vi "main.vi"() -> ()   [LabVIEW 2017]
uses:
  <vilib>/Utility/miscctls.llb/LVRectTypeDef.ctl
  Str_Lam&Sil.ctl
panel:
  out "Wjazd z obu stron":bool
  out "Ilość samochodów na parkingu":dbl
  out "Aktualny stan":T1(ring)
  out "Która brama pierwsza":enum16{"Nikt", "Brama 1", "Brama 2"}(ring)
  in  "output cluster":T2
  out "Brama 2 - kto pierwszy":T3(ring)
  out "Brama 1 - kto pierwszy":T3(ring)
  in  "Ilość miejsc na parkingu":dbl=4.0
  in  "stop":bool
  in  "Dane in":T4
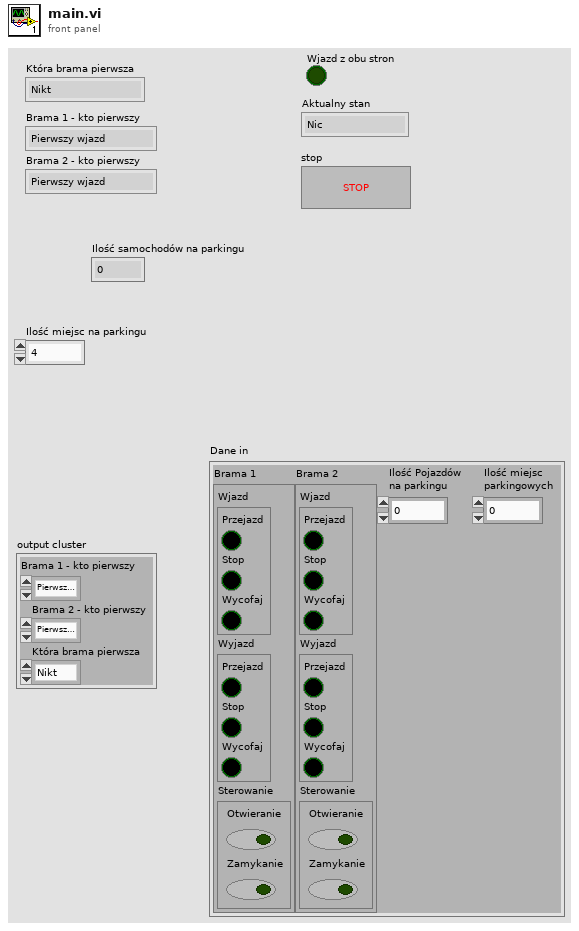
[diagram p1: front panel]
types:
  T1 = enum16{"Nic", "Otwieranie", "Otwarte", "Wjazd", "Wyjazd", "Zamykanie", "Wycofaj", "Blad"}
  T2 = cluster{"Brama 1 - kto pierwszy":enum16{"Pierwszy wjazd", "Nikt", "Pierwszy wyjazd"}, "Brama 2 - kto pierwszy":enum16{"Pierwszy wjazd", "Nikt", "Pierwszy wyjazd"}, "Która brama pierwsza":enum16{"Nikt", "Brama 1", "Brama 2"}}
  T3 = enum16{"Pierwszy wjazd", "Nikt", "Pierwszy wyjazd"}
  T4 = cluster{"Brama 1":cluster{"Wjazd":cluster{"Wjazd Przejazd":bool, "Wjazd Stop":bool, "Wjazd Wycofaj":bool}, "Wyjazd":cluster{"Wjazd Przejazd":bool, "Wjazd Stop":bool, "Wjazd Wycofaj":bool}, "Sterowanie":cluster{"Otwieranie":bool, "Zamykanie":bool}}, "Brama 2":cluster{"Wjazd":cluster{"Wjazd Przejazd":bool, "Wjazd Stop":bool, "Wjazd Wycofaj":bool}, "Wyjazd":cluster{"Wjazd Przejazd":bool, "Wjazd Stop":bool, "Wjazd Wycofaj":bool}, "Sterowanie":cluster{"Otwieranie":bool, "Zamykanie":bool}}, "Ilość Pojazdów \nna parkingu":dbl, "Ilość miejsc \nparkingowych":dbl}
  T5 = typedef "LVRectTypeDef.ctl" = cluster{"Left":i16, "Top":i16, "Right":i16, "Bottom":i16}
  T6 = typedef "Str_Lam&Sil.ctl" = bool
  T7 = cluster{"Wjazd":cluster{"Wjazd Przejazd":T6, "Wjazd Stop":bool, "Wjazd Wycofaj":bool}, "Wyjazd":cluster{"Wjazd Przejazd":bool, "Wjazd Stop":bool, "Wjazd Wycofaj":bool}, "Sterowanie":cluster{"Otwieranie":bool, "Zamykanie":bool}}
  T8 = cluster{"czujnik laserowy \nwjazd":bool, "czujnik laserowy wyjazd":bool, "czujnik laserowy \nbrama zamknięta":bool, "czujnik laserowy \nbrama otwarta":bool}
  T9 = cluster{"Brama 1":cluster{"czujnik laserowy \nwjazd":bool, "czujnik laserowy wyjazd":bool, "czujnik laserowy \nbrama zamknięta":bool, "czujnik laserowy \nbrama otwarta":bool}, "Brama 2":cluster{"czujnik laserowy \nwjazd":bool, "czujnik laserowy wyjazd":bool, "czujnik laserowy \nbrama zamknięta":bool, "czujnik laserowy \nbrama otwarta":bool}}
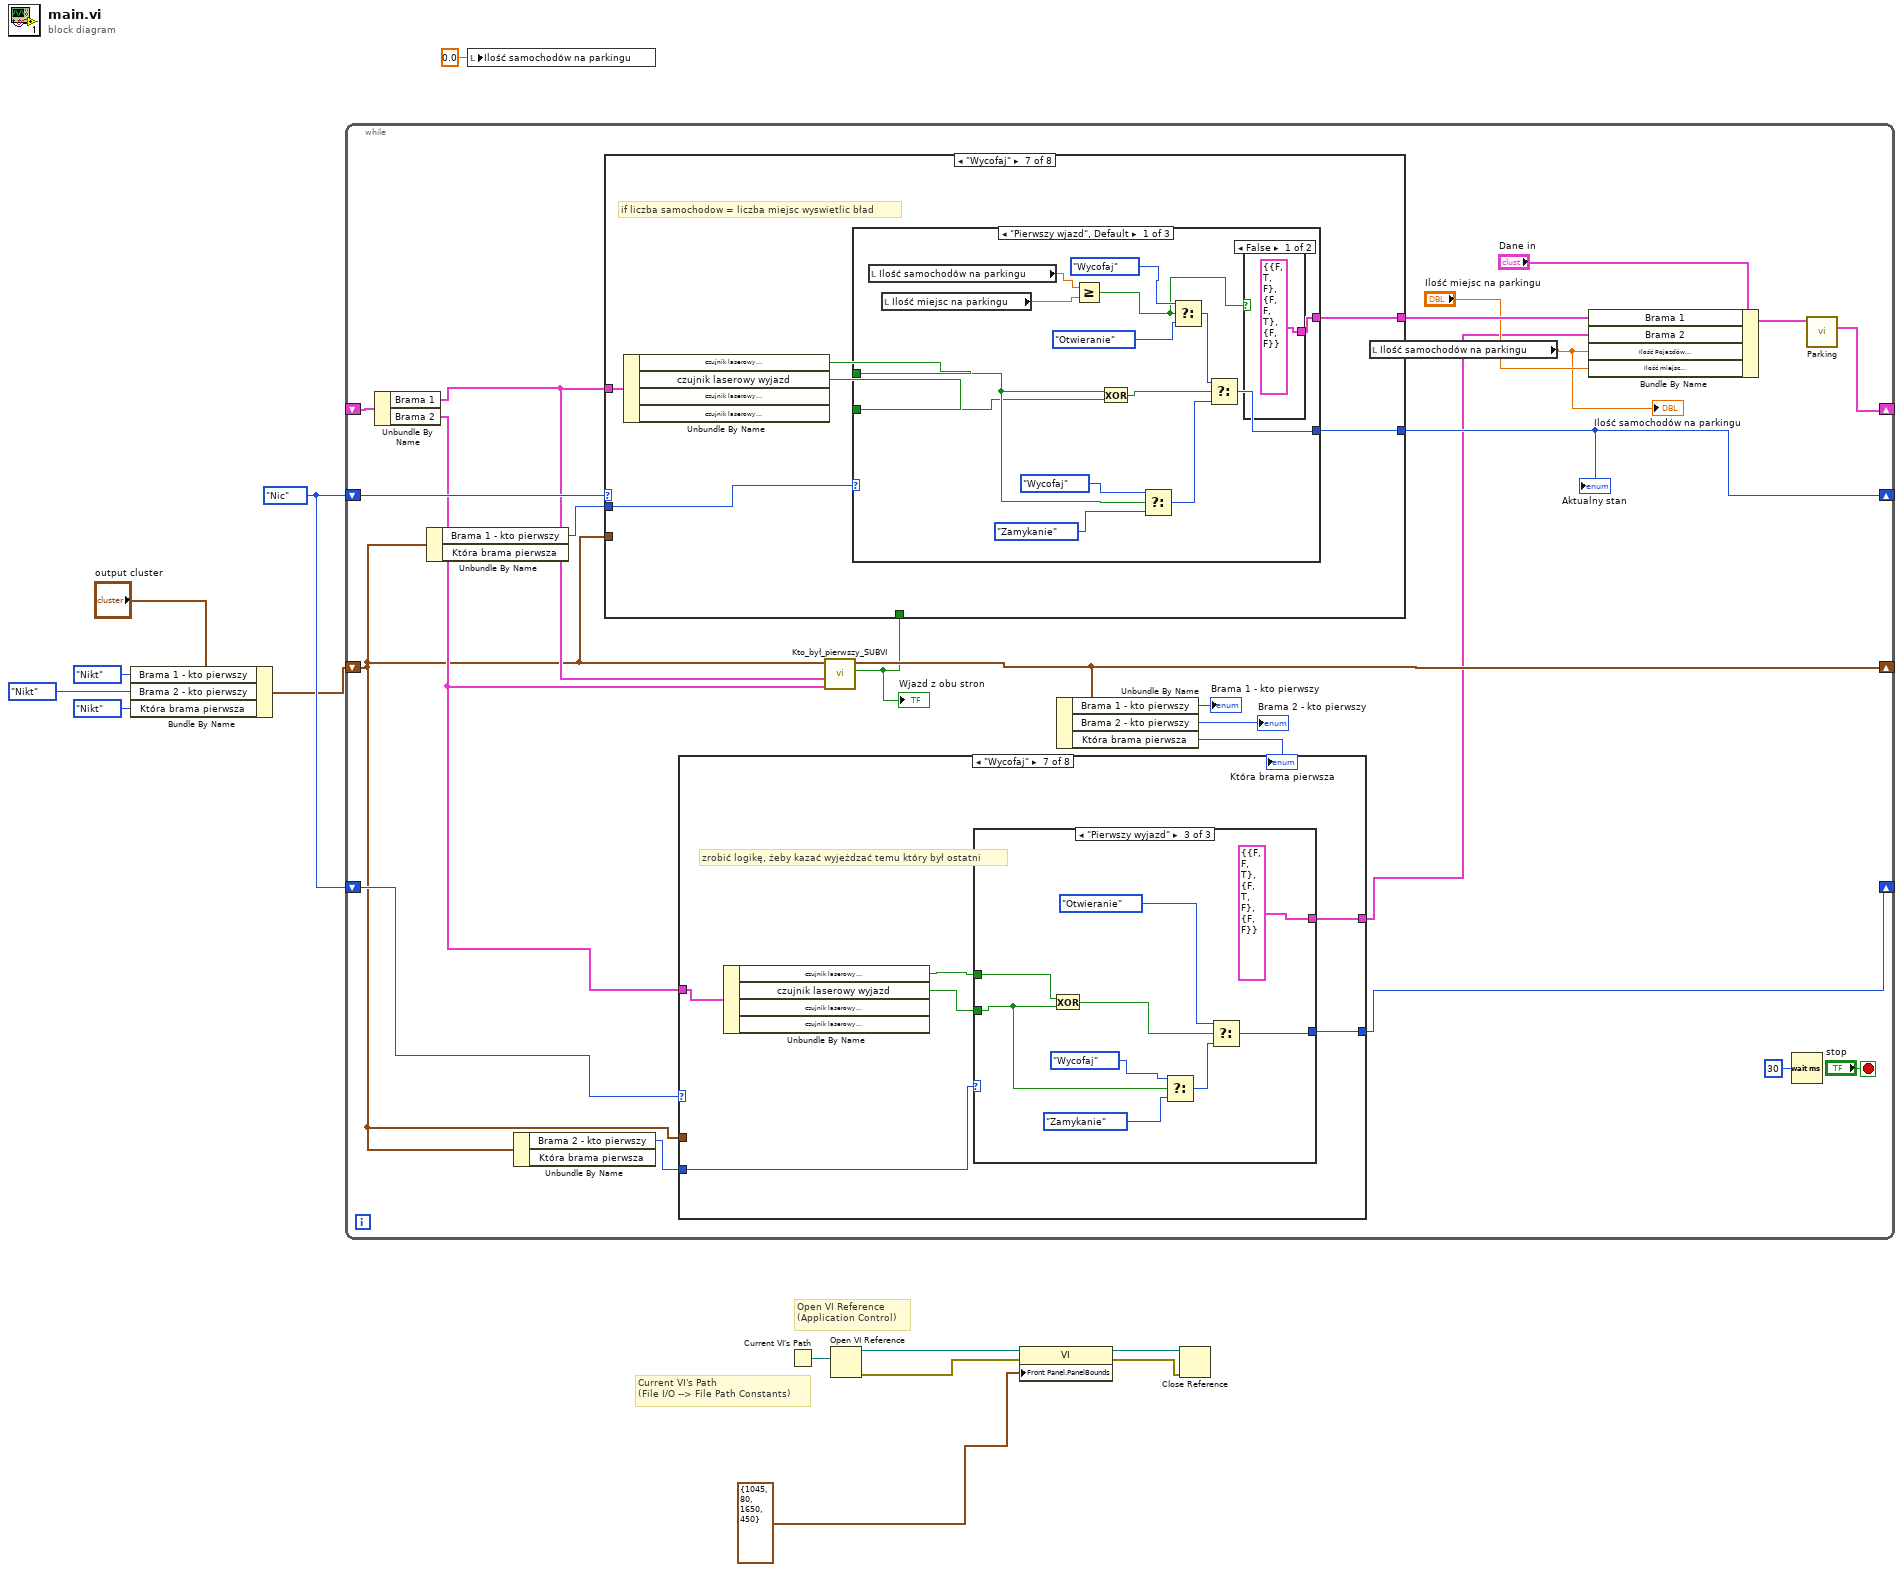
[diagram p0: block diagram]
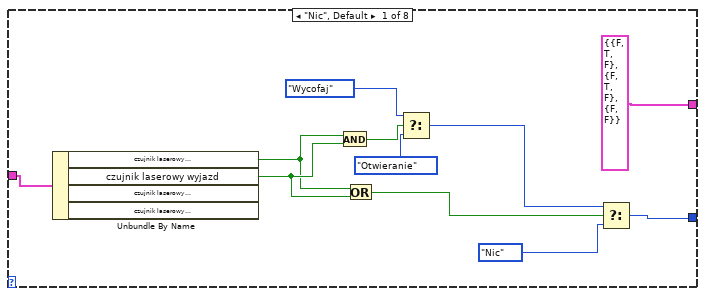
[diagram p2: hidden frame]
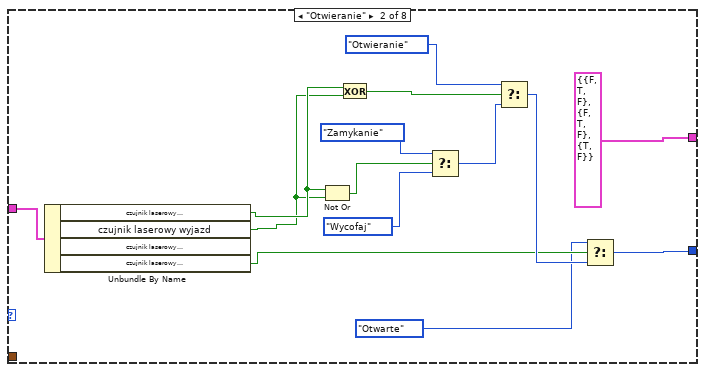
[diagram p3: hidden frame]
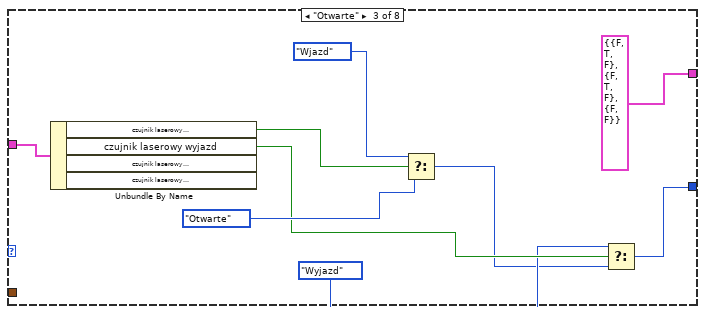
[diagram p4: hidden frame]
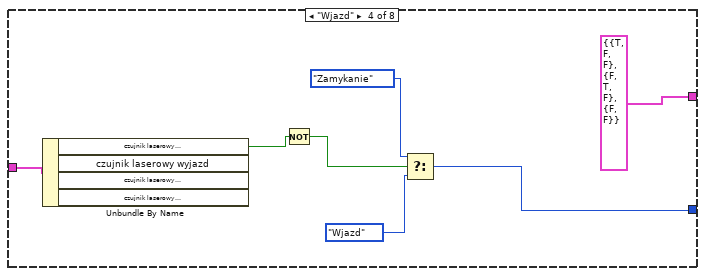
[diagram p5: hidden frame]
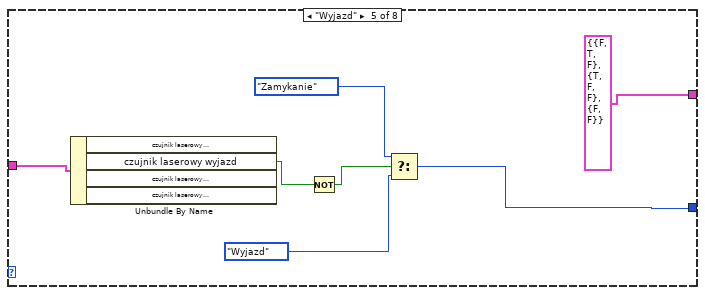
[diagram p6: hidden frame]
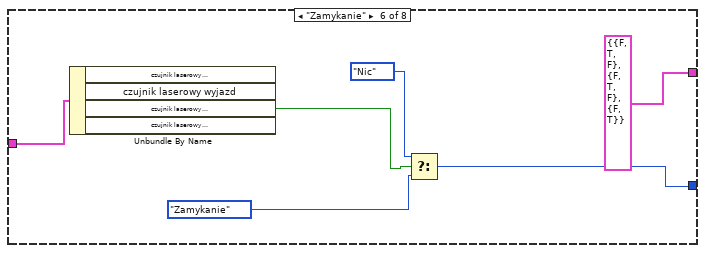
[diagram p7: hidden frame]
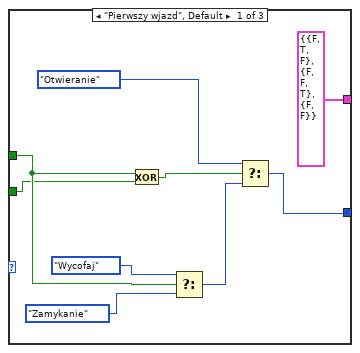
[diagram p8: hidden frame]
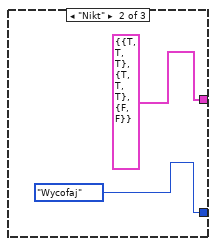
[diagram p9: hidden frame]
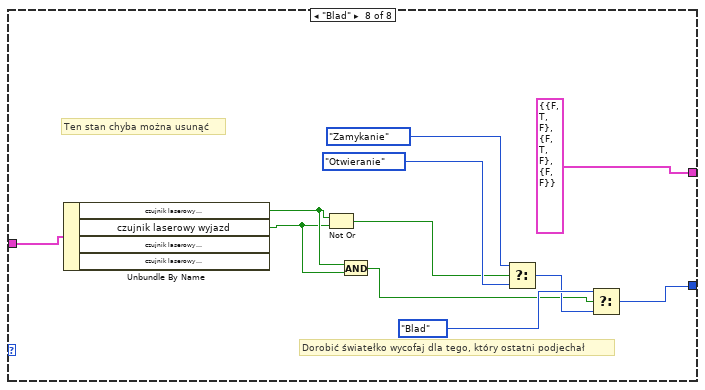
[diagram p10: hidden frame]
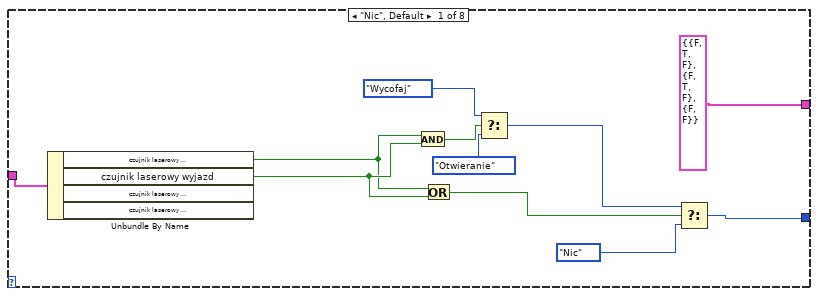
[diagram p11: hidden frame]
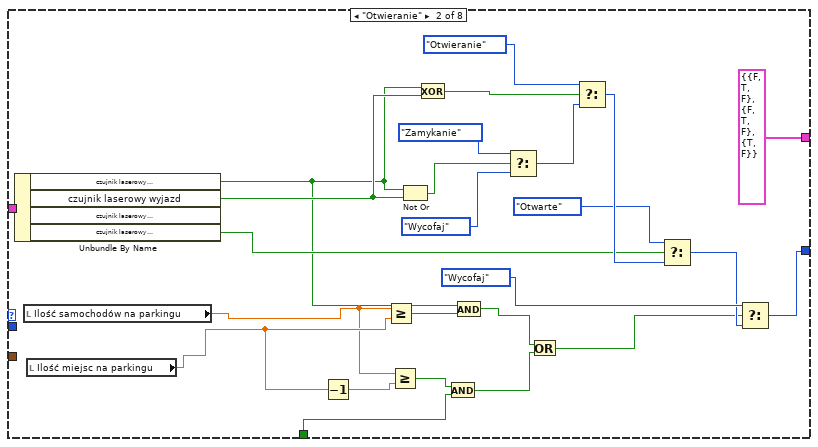
[diagram p12: hidden frame]
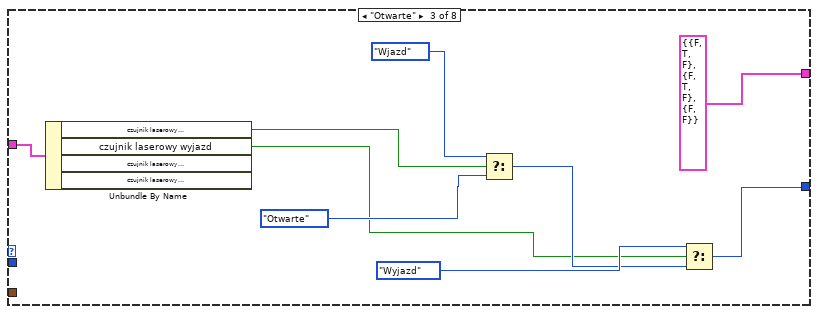
[diagram p13: hidden frame]
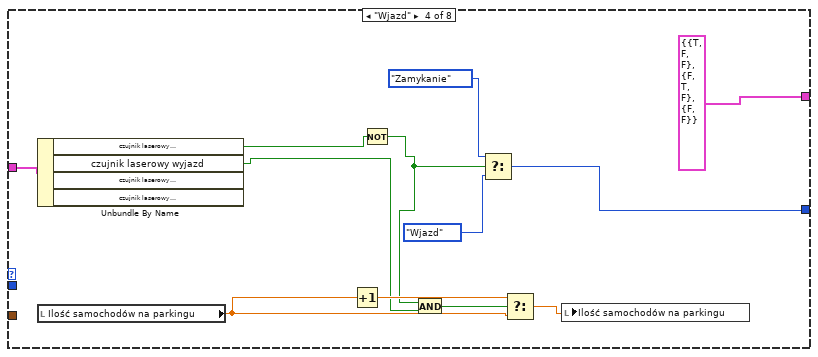
[diagram p14: hidden frame]
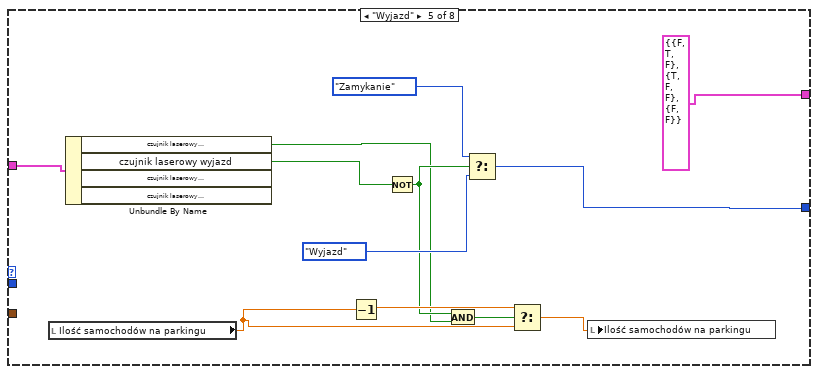
[diagram p15: hidden frame]
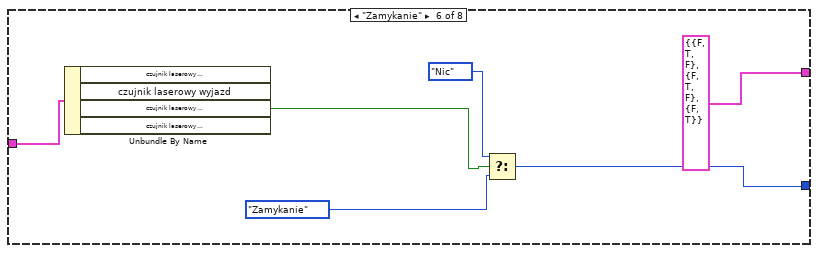
[diagram p16: hidden frame]
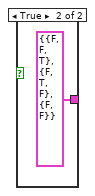
[diagram p17: hidden frame]
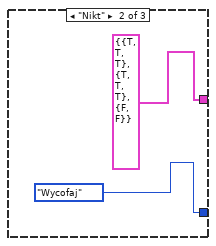
[diagram p18: hidden frame]
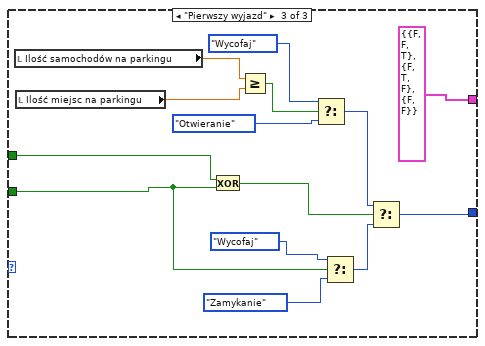
[diagram p19: hidden frame]
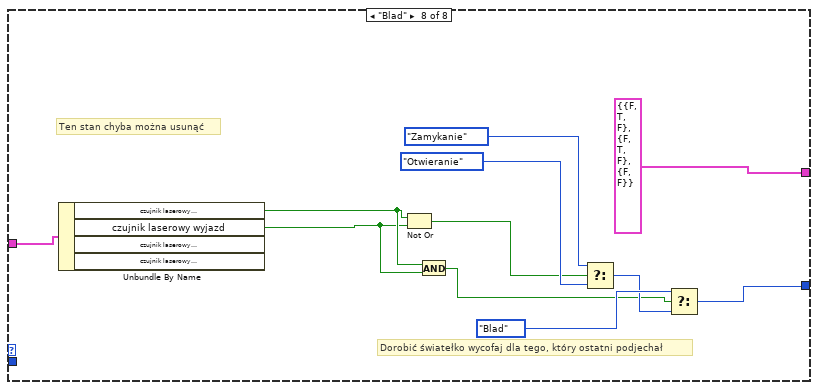
[diagram p20: hidden frame]
diagram:
  w13 = T1."Nic"
  # "Open VI Reference\n(Application Control)"
  # "Current VI's Path\n(File I/O --> File Path Constants)"
  n1 = Bundle By Name(cluster="output cluster", "Brama 1 - kto pierwszy"=T3."Nikt", "Brama 2 - kto pierwszy"=T3."Nikt", "Która brama pierwsza"=enum16{"Nikt", "Brama 1", "Brama 2"}."Nikt") -> (w11:T2)
  n2 = while {
    shift-right: [w34] -> _
    shift-left: _ -> [w35]
    shift-right: [w31] -> _
    shift-left: w13 -> [w29]
    shift-right: [w21] -> _
    shift-left: w13 -> [w20]
    shift-right: [w26] -> _
    shift-left: w11 -> [w18]
    stop <- "stop" stop-if-true
    n3 = Unbundle By Name(w35) -> ("Brama 1"=w27:T8, "Brama 2"=w19:T8)
    n4 = Unbundle By Name(w18) -> ("Brama 1 - kto pierwszy"=w16:T3)  [unwired: 1 out]
    n5 = Unbundle By Name(w18) -> ("Brama 2 - kto pierwszy"=w15:T3)  [unwired: 1 out]
    n6 = case shown="\"Wycofaj\"" w20 {
      tunnel: w19 -> [w40 w62 w63 w76 w81 w88 w97 w127]
      tunnel: [w41 w61 w65 w75 w83 w86 w93 w124] -> w21
      tunnel: [T7 {"Wjazd"={"Wjazd Przejazd"=FALSE, "Wjazd Stop"=TRUE, "Wjazd Wycofaj"=FALSE}, "Wyjazd"={"Wjazd Przejazd"=FALSE, "Wjazd Stop"=TRUE, "Wjazd Wycofaj"=FALSE}, "Sterowanie"={"Otwieranie"=FALSE, "Zamykanie"=FALSE}} ("Brama 1") T7 {"Wjazd"={"Wjazd Przejazd"=FALSE, "Wjazd Stop"=TRUE, "Wjazd Wycofaj"=FALSE}, "Wyjazd"={"Wjazd Przejazd"=FALSE, "Wjazd Stop"=TRUE, "Wjazd Wycofaj"=FALSE}, "Sterowanie"={"Otwieranie"=TRUE, "Zamykanie"=FALSE}} ("Brama 1") T7 {"Wjazd"={"Wjazd Przejazd"=FALSE, "Wjazd Stop"=TRUE, "Wjazd Wycofaj"=FALSE}, "Wyjazd"={"Wjazd Przejazd"=FALSE, "Wjazd Stop"=TRUE, "Wjazd Wycofaj"=FALSE}, "Sterowanie"={"Otwieranie"=FALSE, "Zamykanie"=FALSE}} ("Brama 1") T7 {"Wjazd"={"Wjazd Przejazd"=TRUE, "Wjazd Stop"=FALSE, "Wjazd Wycofaj"=FALSE}, "Wyjazd"={"Wjazd Przejazd"=FALSE, "Wjazd Stop"=TRUE, "Wjazd Wycofaj"=FALSE}, "Sterowanie"={"Otwieranie"=FALSE, "Zamykanie"=FALSE}} ("Brama 1") T7 {"Wjazd"={"Wjazd Przejazd"=FALSE, "Wjazd Stop"=TRUE, "Wjazd Wycofaj"=FALSE}, "Wyjazd"={"Wjazd Przejazd"=TRUE, "Wjazd Stop"=FALSE, "Wjazd Wycofaj"=FALSE}, "Sterowanie"={"Otwieranie"=FALSE, "Zamykanie"=FALSE}} ("Brama 1") T7 {"Wjazd"={"Wjazd Przejazd"=FALSE, "Wjazd Stop"=TRUE, "Wjazd Wycofaj"=FALSE}, "Wyjazd"={"Wjazd Przejazd"=FALSE, "Wjazd Stop"=TRUE, "Wjazd Wycofaj"=FALSE}, "Sterowanie"={"Otwieranie"=FALSE, "Zamykanie"=TRUE}} ("Brama 1") w94 T7 {"Wjazd"={"Wjazd Przejazd"=FALSE, "Wjazd Stop"=TRUE, "Wjazd Wycofaj"=FALSE}, "Wyjazd"={"Wjazd Przejazd"=FALSE, "Wjazd Stop"=TRUE, "Wjazd Wycofaj"=FALSE}, "Sterowanie"={"Otwieranie"=FALSE, "Zamykanie"=FALSE}} ("Brama 1")] -> w22
      tunnel: w18 -> [_ _ _ _ _ _ _ _]
      tunnel: w15 -> [_ _ _ _ _ _ w92 _]
      frame "Nic", Default {
        n7 = Unbundle By Name(w40) -> ("czujnik laserowy \nwjazd"=w38:bool, "czujnik laserowy wyjazd"=w46:bool)  [unwired: 2 out]
        n8 = And(x=w38, y=w46) -> (x .and. y?=w48:bool)
        n9 = Or(x=w38, y=w46) -> (x .or. y?=w45:bool)
        n10 = Select(t=T1."Wycofaj", s=w48, f=T1."Otwieranie") -> (s? t:f=w44:T1)
        n11 = Select(t=w44, s=w45, f=T1."Nic") -> (s? t:f=w41:T1)
      }
      frame "Otwieranie" {
        n12 = Unbundle By Name(w62) -> ("czujnik laserowy \nwjazd"=w52:bool, "czujnik laserowy wyjazd"=w51:bool, "czujnik laserowy \nbrama otwarta"=w58:bool)  [unwired: 1 out]
        n13 = Not Or(1:w51, 2:w52) -> (0:w56:bool)
        n14 = Exclusive Or(1:w51, 2:w52) -> (0:w53:bool)
        n15 = Select(t=T1."Zamykanie", s=w56, f=T1."Wycofaj") -> (s? t:f=w49:T1)
        n16 = Select(t=T1."Otwieranie", s=w53, f=w49) -> (s? t:f=w59:T1)
        n17 = Select(t=T1."Otwarte", s=w58, f=w59) -> (s? t:f=w61:T1)
      }
      frame "Otwarte" {
        n18 = Unbundle By Name(w63) -> ("czujnik laserowy \nwjazd"=w69:bool, "czujnik laserowy wyjazd"=w68:bool)  [unwired: 2 out]
        n19 = Select(t=T1."Wjazd", s=w69, f=T1."Otwarte") -> (s? t:f=w66:T1)
        n20 = Select(t=T1."Wyjazd", s=w68, f=w66) -> (s? t:f=w65:T1)
      }
      frame "Wjazd" {
        n21 = Unbundle By Name(w76) -> ("czujnik laserowy \nwjazd"=w73:bool)  [unwired: 3 out]
        n22 = Not(x=w73) -> (.not. x?=w72:bool)
        n23 = Select(t=T1."Zamykanie", s=w72, f=T1."Wjazd") -> (s? t:f=w75:T1)
      }
      frame "Wyjazd" {
        n24 = Unbundle By Name(w81) -> ("czujnik laserowy wyjazd"=w80:bool)  [unwired: 3 out]
        n25 = Not(x=w80) -> (.not. x?=w79:bool)
        n26 = Select(t=T1."Zamykanie", s=w79, f=T1."Wyjazd") -> (s? t:f=w83:T1)
      }
      frame "Zamykanie" {
        n27 = Unbundle By Name(w88) -> ("czujnik laserowy \nbrama zamknięta"=w87:bool)  [unwired: 3 out]
        n28 = Select(t=T1."Nic", s=w87, f=T1."Zamykanie") -> (s? t:f=w86:T1)
      }
      frame "Wycofaj" {
        # "zrobić logikę, żeby kazać wyjeżdzać temu który był ostatni"
        n29 = Unbundle By Name(w97) -> ("czujnik laserowy \nwjazd"=w95:bool, "czujnik laserowy wyjazd"=w96:bool)  [unwired: 2 out]
        n30 = case shown="\"Pierwszy wyjazd\"" w92 {
          tunnel: w96 -> [w98 _ w109]
          tunnel: w95 -> [w99 _ w115]
          tunnel: [T7 {"Wjazd"={"Wjazd Przejazd"=FALSE, "Wjazd Stop"=TRUE, "Wjazd Wycofaj"=FALSE}, "Wyjazd"={"Wjazd Przejazd"=FALSE, "Wjazd Stop"=FALSE, "Wjazd Wycofaj"=TRUE}, "Sterowanie"={"Otwieranie"=FALSE, "Zamykanie"=FALSE}} ("Brama 1") T7 {"Wjazd"={"Wjazd Przejazd"=TRUE, "Wjazd Stop"=TRUE, "Wjazd Wycofaj"=TRUE}, "Wyjazd"={"Wjazd Przejazd"=TRUE, "Wjazd Stop"=TRUE, "Wjazd Wycofaj"=TRUE}, "Sterowanie"={"Otwieranie"=FALSE, "Zamykanie"=FALSE}} ("Brama 1") T7 {"Wjazd"={"Wjazd Przejazd"=FALSE, "Wjazd Stop"=FALSE, "Wjazd Wycofaj"=TRUE}, "Wyjazd"={"Wjazd Przejazd"=FALSE, "Wjazd Stop"=TRUE, "Wjazd Wycofaj"=FALSE}, "Sterowanie"={"Otwieranie"=FALSE, "Zamykanie"=FALSE}} ("Brama 1")] -> w94
          tunnel: [w104 T1."Wycofaj" w116] -> w93
          frame "Pierwszy wjazd", Default {
            n31 = Exclusive Or(1:w98, 2:w99) -> (0:w100:bool)
            n32 = Select(t=T1."Wycofaj", s=w99, f=T1."Zamykanie") -> (s? t:f=w101:T1)
            n33 = Select(t=T1."Otwieranie", s=w100, f=w101) -> (s? t:f=w104:T1)
          }
          frame "Nikt" {
          }
          frame "Pierwszy wyjazd" {
            n34 = Exclusive Or(1:w109, 2:w115) -> (0:w114:bool)
            n35 = Select(t=T1."Wycofaj", s=w109, f=T1."Zamykanie") -> (s? t:f=w110:T1)
            n36 = Select(t=T1."Otwieranie", s=w114, f=w110) -> (s? t:f=w116:T1)
          }
        }
      }
      frame "Blad" {
        # "Ten stan chyba można usunąć"
        # "Dorobić światełko wycofaj dla tego, który ostatni podjechał"
        n37 = Unbundle By Name(w127) -> ("czujnik laserowy \nwjazd"=w120:bool, "czujnik laserowy wyjazd"=w119:bool)  [unwired: 2 out]
        n38 = Not Or(1:w119, 2:w120) -> (0:w121:bool)
        n39 = And(x=w120, y=w119) -> (x .and. y?=w118:bool)
        n40 = Select(t=T1."Zamykanie", s=w121, f=T1."Otwieranie") -> (s? t:f=w122:T1)
        n41 = Select(t=T1."Blad", s=w118, f=w122) -> (s? t:f=w124:T1)
      }
    }
    n42 = call "Kto_był_pierwszy_SUBVI.vi"("Brama 2"=w19, "Brama 1"=w27, "Wejscie"=w18) -> ("Wjazd z obu stron"=w14:bool, "output cluster"=w26:T2)  [unwired: 5 in]
    "Wjazd z obu stron" <- w14
    n43 = case shown="\"Wycofaj\"" w29 {
      tunnel: w27 -> [w131 w164 w167 w183 w193 w200 w209 w251]
      tunnel: [w132 w151 w169 w182 w195 w198 w205 w248] -> w31
      tunnel: [T7 {"Wjazd"={"Wjazd Przejazd"=FALSE, "Wjazd Stop"=TRUE, "Wjazd Wycofaj"=FALSE}, "Wyjazd"={"Wjazd Przejazd"=FALSE, "Wjazd Stop"=TRUE, "Wjazd Wycofaj"=FALSE}, "Sterowanie"={"Otwieranie"=FALSE, "Zamykanie"=FALSE}} ("Brama 1") T7 {"Wjazd"={"Wjazd Przejazd"=FALSE, "Wjazd Stop"=TRUE, "Wjazd Wycofaj"=FALSE}, "Wyjazd"={"Wjazd Przejazd"=FALSE, "Wjazd Stop"=TRUE, "Wjazd Wycofaj"=FALSE}, "Sterowanie"={"Otwieranie"=TRUE, "Zamykanie"=FALSE}} ("Brama 1") T7 {"Wjazd"={"Wjazd Przejazd"=FALSE, "Wjazd Stop"=TRUE, "Wjazd Wycofaj"=FALSE}, "Wyjazd"={"Wjazd Przejazd"=FALSE, "Wjazd Stop"=TRUE, "Wjazd Wycofaj"=FALSE}, "Sterowanie"={"Otwieranie"=FALSE, "Zamykanie"=FALSE}} ("Brama 1") T7 {"Wjazd"={"Wjazd Przejazd"=TRUE, "Wjazd Stop"=FALSE, "Wjazd Wycofaj"=FALSE}, "Wyjazd"={"Wjazd Przejazd"=FALSE, "Wjazd Stop"=TRUE, "Wjazd Wycofaj"=FALSE}, "Sterowanie"={"Otwieranie"=FALSE, "Zamykanie"=FALSE}} ("Brama 1") T7 {"Wjazd"={"Wjazd Przejazd"=FALSE, "Wjazd Stop"=TRUE, "Wjazd Wycofaj"=FALSE}, "Wyjazd"={"Wjazd Przejazd"=TRUE, "Wjazd Stop"=FALSE, "Wjazd Wycofaj"=FALSE}, "Sterowanie"={"Otwieranie"=FALSE, "Zamykanie"=FALSE}} ("Brama 1") T7 {"Wjazd"={"Wjazd Przejazd"=FALSE, "Wjazd Stop"=TRUE, "Wjazd Wycofaj"=FALSE}, "Wyjazd"={"Wjazd Przejazd"=FALSE, "Wjazd Stop"=TRUE, "Wjazd Wycofaj"=FALSE}, "Sterowanie"={"Otwieranie"=FALSE, "Zamykanie"=TRUE}} ("Brama 1") w206 T7 {"Wjazd"={"Wjazd Przejazd"=FALSE, "Wjazd Stop"=TRUE, "Wjazd Wycofaj"=FALSE}, "Wyjazd"={"Wjazd Przejazd"=FALSE, "Wjazd Stop"=TRUE, "Wjazd Wycofaj"=FALSE}, "Sterowanie"={"Otwieranie"=FALSE, "Zamykanie"=FALSE}} ("Brama 1")] -> w30
      tunnel: w18 -> [_ _ _ _ _ _ _ _]
      tunnel: w16 -> [_ _ _ _ _ _ w204 _]
      tunnel: w14 -> [_ w143 _ _ _ _ _ _]
      frame "Nic", Default {
        n44 = Unbundle By Name(w131) -> ("czujnik laserowy \nwjazd"=w129:bool, "czujnik laserowy wyjazd"=w137:bool)  [unwired: 2 out]
        n45 = And(x=w129, y=w137) -> (x .and. y?=w139:bool)
        n46 = Or(x=w129, y=w137) -> (x .or. y?=w136:bool)
        n47 = Select(t=T1."Wycofaj", s=w139, f=T1."Otwieranie") -> (s? t:f=w135:T1)
        n48 = Select(t=w135, s=w136, f=T1."Nic") -> (s? t:f=w132:T1)
      }
      frame "Otwieranie" {
        n49 = Unbundle By Name(w164) -> ("czujnik laserowy \nwjazd"=w148:bool, "czujnik laserowy wyjazd"=w155:bool, "czujnik laserowy \nbrama otwarta"=w161:bool)  [unwired: 1 out]
        n50 = local read "Ilość samochodów na parkingu"() -> (w145:dbl)
        n51 = local read "Ilość miejsc na parkingu"() -> (w147:dbl)
        n52 = Decrement(x=w147) -> (x-1=w146:dbl)
        n53 = Greater Or Equal?(x=w145, y=w147) -> (x >= y?=w149:bool)
        n54 = Greater Or Equal?(x=w145, y=w146) -> (x >= y?=w144:bool)
        n55 = Not Or(1:w155, 2:w148) -> (0:w159:bool)
        n56 = Exclusive Or(1:w155, 2:w148) -> (0:w156:bool)
        n57 = And(x=w144, y=w143) -> (x .and. y?=w142:bool)
        n58 = And(x=w148, y=w149) -> (x .and. y?=w141:bool)
        n59 = Select(t=T1."Zamykanie", s=w159, f=T1."Wycofaj") -> (s? t:f=w153:T1)
        n60 = Or(x=w141, y=w142) -> (x .or. y?=w140:bool)
        n61 = Select(t=T1."Otwieranie", s=w156, f=w153) -> (s? t:f=w162:T1)
        n62 = Select(t=T1."Otwarte", s=w161, f=w162) -> (s? t:f=w150:T1)
        n63 = Select(t=T1."Wycofaj", s=w140, f=w150) -> (s? t:f=w151:T1)
      }
      frame "Otwarte" {
        n64 = Unbundle By Name(w167) -> ("czujnik laserowy \nwjazd"=w166:bool, "czujnik laserowy wyjazd"=w165:bool)  [unwired: 2 out]
        n65 = Select(t=T1."Wjazd", s=w166, f=T1."Otwarte") -> (s? t:f=w170:T1)
        n66 = Select(t=T1."Wyjazd", s=w165, f=w170) -> (s? t:f=w169:T1)
      }
      frame "Wjazd" {
        n67 = Unbundle By Name(w183) -> ("czujnik laserowy \nwjazd"=w180:bool, "czujnik laserowy wyjazd"=w174:bool)  [unwired: 2 out]
        n68 = local read "Ilość samochodów na parkingu"() -> (w178:dbl)
        n69 = Increment(x=w178) -> (x+1=w179:dbl)
        n70 = Not(x=w180) -> (.not. x?=w175:bool)
        n71 = And(x=w175, y=w174) -> (x .and. y?=w176:bool)
        n72 = Select(t=T1."Zamykanie", s=w175, f=T1."Wjazd") -> (s? t:f=w182:T1)
        n73 = Select(t=w179, s=w176, f=w178) -> (s? t:f=w177:dbl)
        n74 = local write "Ilość samochodów na parkingu"(w177) -> ()
      }
      frame "Wyjazd" {
        n75 = local read "Ilość samochodów na parkingu"() -> (w190:dbl)
        n76 = Unbundle By Name(w193) -> ("czujnik laserowy \nwjazd"=w186:bool, "czujnik laserowy wyjazd"=w192:bool)  [unwired: 2 out]
        n77 = Decrement(x=w190) -> (x-1=w191:dbl)
        n78 = Not(x=w192) -> (.not. x?=w187:bool)
        n79 = And(x=w187, y=w186) -> (x .and. y?=w188:bool)
        n80 = Select(t=T1."Zamykanie", s=w187, f=T1."Wyjazd") -> (s? t:f=w195:T1)
        n81 = Select(t=w191, s=w188, f=w190) -> (s? t:f=w189:dbl)
        n82 = local write "Ilość samochodów na parkingu"(w189) -> ()
      }
      frame "Zamykanie" {
        n83 = Unbundle By Name(w200) -> ("czujnik laserowy \nbrama zamknięta"=w199:bool)  [unwired: 3 out]
        n84 = Select(t=T1."Nic", s=w199, f=T1."Zamykanie") -> (s? t:f=w198:T1)
      }
      frame "Wycofaj" {
        # "if liczba samochodow = liczba miejsc wyswietlic bład"
        n85 = Unbundle By Name(w209) -> ("czujnik laserowy \nwjazd"=w207:bool, "czujnik laserowy wyjazd"=w208:bool)  [unwired: 2 out]
        n86 = case shown="\"Pierwszy wjazd\", Default" w204 {
          tunnel: w208 -> [w217 _ w234]
          tunnel: w207 -> [w218 _ w239]
          tunnel: [w211 T7 {"Wjazd"={"Wjazd Przejazd"=TRUE, "Wjazd Stop"=TRUE, "Wjazd Wycofaj"=TRUE}, "Wyjazd"={"Wjazd Przejazd"=TRUE, "Wjazd Stop"=TRUE, "Wjazd Wycofaj"=TRUE}, "Sterowanie"={"Otwieranie"=FALSE, "Zamykanie"=FALSE}} ("Brama 1") T7 {"Wjazd"={"Wjazd Przejazd"=FALSE, "Wjazd Stop"=FALSE, "Wjazd Wycofaj"=TRUE}, "Wyjazd"={"Wjazd Przejazd"=FALSE, "Wjazd Stop"=TRUE, "Wjazd Wycofaj"=FALSE}, "Sterowanie"={"Otwieranie"=FALSE, "Zamykanie"=FALSE}} ("Brama 1")] -> w206
          tunnel: [w223 T1."Wycofaj" w240] -> w205
          frame "Pierwszy wjazd", Default {
            n87 = local read "Ilość samochodów na parkingu"() -> (w216:dbl)
            n88 = local read "Ilość miejsc na parkingu"() -> (w215:dbl)
            n89 = Greater Or Equal?(x=w216, y=w215) -> (x >= y?=w210:bool)
            n90 = Exclusive Or(1:w217, 2:w218) -> (0:w219:bool)
            n91 = Select(t=T1."Wycofaj", s=w218, f=T1."Zamykanie") -> (s? t:f=w220:T1)
            n92 = Select(t=T1."Wycofaj", s=w210, f=T1."Otwieranie") -> (s? t:f=w212:T1)
            n93 = Select(t=w212, s=w219, f=w220) -> (s? t:f=w223:T1)
            n94 = case shown="False" w210 {
              tunnel: [T7 {"Wjazd"={"Wjazd Przejazd"=FALSE, "Wjazd Stop"=TRUE, "Wjazd Wycofaj"=FALSE}, "Wyjazd"={"Wjazd Przejazd"=FALSE, "Wjazd Stop"=FALSE, "Wjazd Wycofaj"=TRUE}, "Sterowanie"={"Otwieranie"=FALSE, "Zamykanie"=FALSE}} ("Brama 1") T7 {"Wjazd"={"Wjazd Przejazd"=FALSE, "Wjazd Stop"=FALSE, "Wjazd Wycofaj"=TRUE}, "Wyjazd"={"Wjazd Przejazd"=FALSE, "Wjazd Stop"=TRUE, "Wjazd Wycofaj"=FALSE}, "Sterowanie"={"Otwieranie"=FALSE, "Zamykanie"=FALSE}} ("Brama 1")] -> w211
              frame False {
              }
              frame True {
              }
            }
          }
          frame "Nikt" {
          }
          frame "Pierwszy wyjazd" {
            n95 = local read "Ilość samochodów na parkingu"() -> (w229:dbl)
            n96 = local read "Ilość miejsc na parkingu"() -> (w230:dbl)
            n97 = Exclusive Or(1:w234, 2:w239) -> (0:w238:bool)
            n98 = Greater Or Equal?(x=w229, y=w230) -> (x >= y?=w228:bool)
            n99 = Select(t=T1."Wycofaj", s=w228, f=T1."Otwieranie") -> (s? t:f=w232:T1)
            n100 = Select(t=T1."Wycofaj", s=w234, f=T1."Zamykanie") -> (s? t:f=w235:T1)
            n101 = Select(t=w232, s=w238, f=w235) -> (s? t:f=w240:T1)
          }
        }
      }
      frame "Blad" {
        # "Ten stan chyba można usunąć"
        # "Dorobić światełko wycofaj dla tego, który ostatni podjechał"
        n102 = Unbundle By Name(w251) -> ("czujnik laserowy \nwjazd"=w244:bool, "czujnik laserowy wyjazd"=w243:bool)  [unwired: 2 out]
        n103 = Not Or(1:w243, 2:w244) -> (0:w245:bool)
        n104 = And(x=w244, y=w243) -> (x .and. y?=w242:bool)
        n105 = Select(t=T1."Zamykanie", s=w245, f=T1."Otwieranie") -> (s? t:f=w246:T1)
        n106 = Select(t=T1."Blad", s=w242, f=w246) -> (s? t:f=w248:T1)
      }
    }
    "Aktualny stan" <- w31
    n107 = Unbundle By Name(w26) -> ("Brama 1 - kto pierwszy"=→"Brama 1 - kto pierwszy":T3, "Brama 2 - kto pierwszy"=→"Brama 2 - kto pierwszy":T3, "Która brama pierwsza"=→"Która brama pierwsza":enum16{"Nikt", "Brama 1", "Brama 2"})
    n108 = local read "Ilość samochodów na parkingu"() -> (w17:dbl)
    "Ilość samochodów na parkingu" <- w17
    n109 = Bundle By Name(cluster="Dane in", "Brama 1"=w30, "Brama 2"=w22, "Ilość Pojazdów \nna parkingu"=w17, "Ilość miejsc \nparkingowych"="Ilość miejsc na parkingu") -> (w32:T4)
    n110 = Wait (ms)(milliseconds to wait=u32 30) -> ()  [unwired: 1 out]
    n111 = call "Parking.vi"("Dane in"=w32) -> ("Dane out"=w34:T9)  [unwired: 9 in, 1 out]
  }
  n112 = local write "Ilość samochodów na parkingu"(0.0 ("Ilość samochodów na parkingu")) -> ()
  n113 = Current VI's Path() -> (path=w3:path)
  n114 = Open VI Reference(vi path=w3) -> (vi reference=w4:refnum<vi>, error out=w5:errorcluster)  [unwired: 5 in]
  n115 = property class="VI"(reference=w4, error in=w5, "Front Panel.PanelBounds"=T5 {"Left"=1045, "Top"=80, "Right"=1650, "Bottom"=450} ("Desired Front Panel Coordinates")) -> (reference out=w6:refnum<vi>, error out=w7:errorcluster)
  n116 = Close Reference(reference=w6, error in (no error)=w7) -> ()  [unwired: 1 out]
